vi "Datasheet Build TDMS Path.vi"(3 "Serial Number (\"\")":string, 4 "Model Number (\"\")":string, 5 "Test Type (\"\")":string) -> (2 "Path":path)   [LabVIEW 2011]
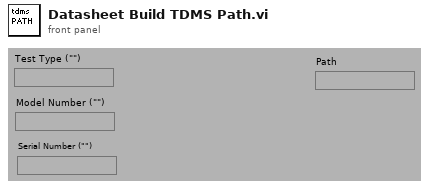
[diagram p1: front panel]
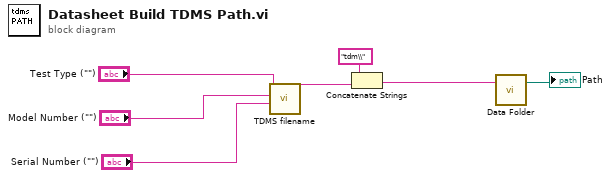
[diagram p0: block diagram]
diagram:
  n1 = call "TDMS filename.vi"("Serial Number"="Serial Number (\"\")", "Model Number"="Model Number (\"\")", "Test Type"="Test Type (\"\")") -> ("Filename"=w4:string)  [unwired: 8 out]
  n2 = Concatenate Strings("tdm\\", w4) -> (w6:string)
  n3 = call "Data Folder.vi"("Relative Path (\"\" - Folder)"=w6) -> ("Data Folder"=→"Path":path)  [unwired: 2 in]
